vi "Flush Q.vi"(7 "Q Ref In":refnum<queue>, 8 "error in":errorcluster) -> (0 "error out":errorcluster, 3 "Remaining Elements":T1[](array[typedef]), 5 "Q Ref Out":refnum<queue>)   [LabVIEW 2025, in "Q Wrappers.lvlib"]
uses:
  Q Wrappers.lvlib
  Q Packet.ctl
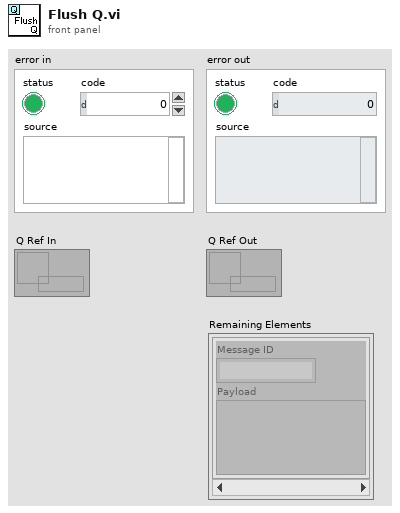
[diagram p1: front panel]
types:
  T1 = typedef "Q Packet.ctl" = cluster{"Message ID":string, "Payload":variant}
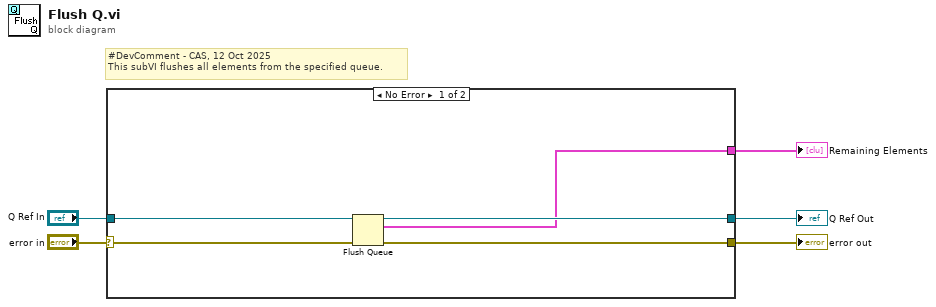
[diagram p0: block diagram]
diagram:
  # "#DevComment - CAS, 12 Oct 2025\nThis subVI flushes all elements from the specified queue."
  n1 = case shown="No Error" "error in" {
    selector: "error in" -> [w10 w12]
    tunnel: [w9 w12] -> w4
    tunnel: [w8 w11] -> w3
    tunnel: "Q Ref In" -> [w7 w11]
    tunnel: [w6 _] -> w1
    frame No Error {
      n2 = Flush Queue(queue=w7, error in (no error)=w10) -> (queue out=w8:refnum<queue>, remaining elements=w6:T1[], error out=w9:errorcluster)
    }
    frame Error {
    }
  }
  "error out" <- w4
  "Q Ref Out" <- w3
  "Remaining Elements" <- w1
